vi "IsReadyToKick.vi"(0 "KickToSkill in":refnum<class "KickToSkill.lvclass">, 1 "KickEps":dbl, 2 "KickRange":dbl, 5 "Game":refnum<class "Game.lvclass">, 7 "Target":dbl[](array[numeric]), 9 "Robot":refnum<class "Robot.lvclass">, 11 "error in (no error)":errorcluster, 12 "MinDistToKick":dbl, 13 "KickingAngle":dbl, 14 "DistToKickingAngle":dbl) -> (4 "KickToSkill out":refnum<class "KickToSkill.lvclass">, 6 "CanKick?":bool, 15 "error out":errorcluster)   [LabVIEW 2020, in "KickToSkill.lvclass"]
uses:
  KickToSkill.lvclass
  Game_class/Game.lvclass
  Robot_class/Robot.lvclass
  Utilities_class/Utilities.lvclass
  Object_class/Object.lvclass/Object.ctl
  Robot_class/Robot.lvclass/Robot.ctl
  Game_class/Game.lvclass/Game.ctl
  <vilib>/Analysis/coordinate.llb/2D Cartesian Coordinate Rotation (Scalar).vi
  Game_class/Read BallRef.vi
  Object_class/Read x.vi
  Object_class/Read y.vi
  Robot_class/Read orientation.vi
  Ball_class/Ball.lvclass
  <vilib>/Analysis/NI_AALPro.lvlib
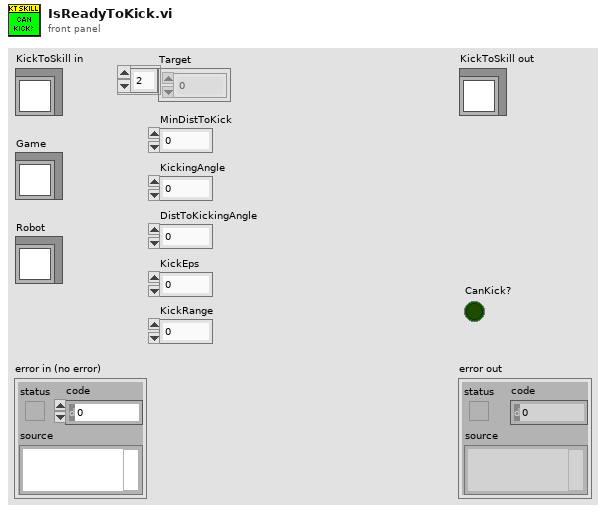
[diagram p1: front panel]
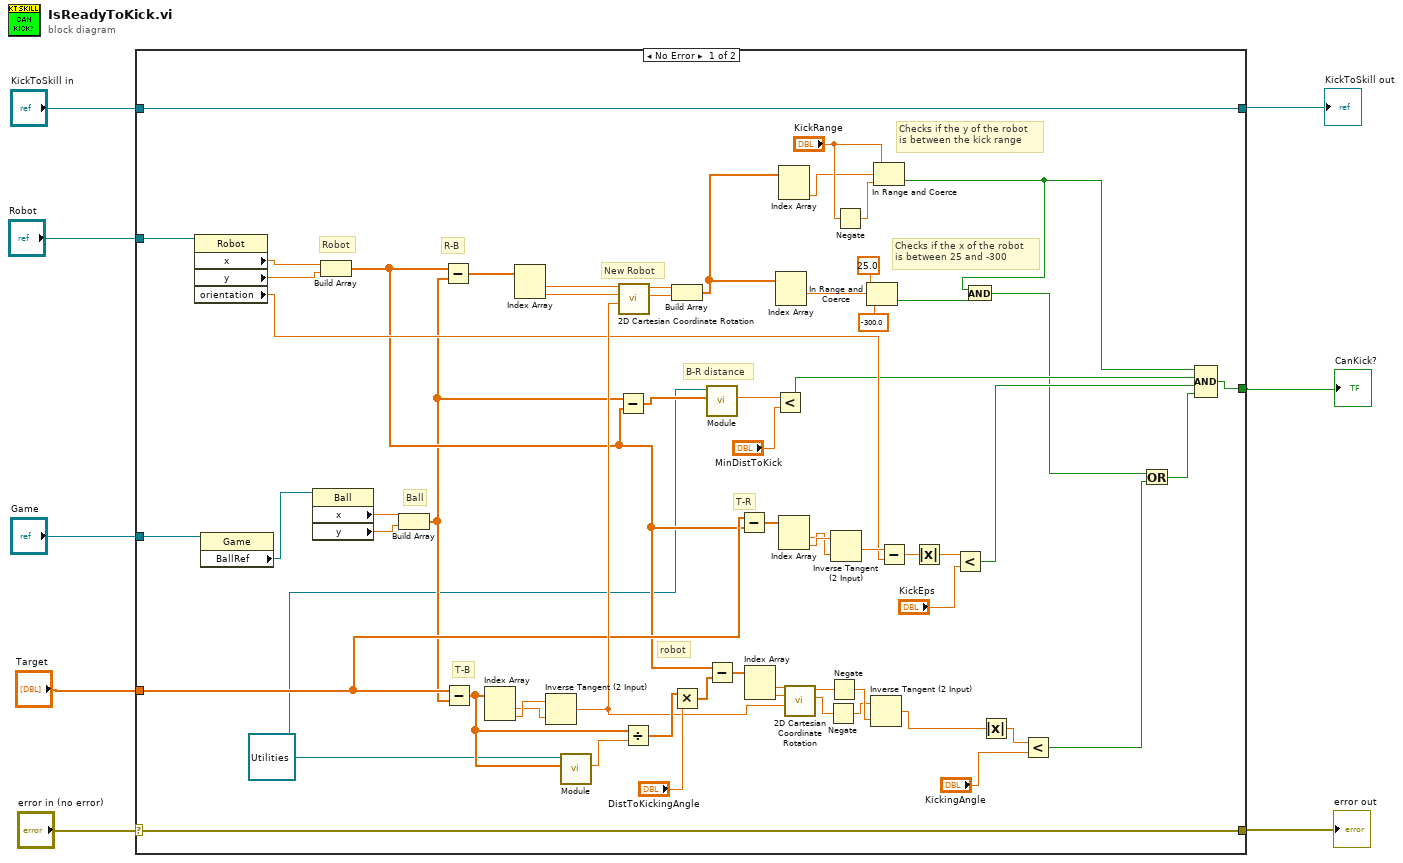
[diagram p0: block diagram]
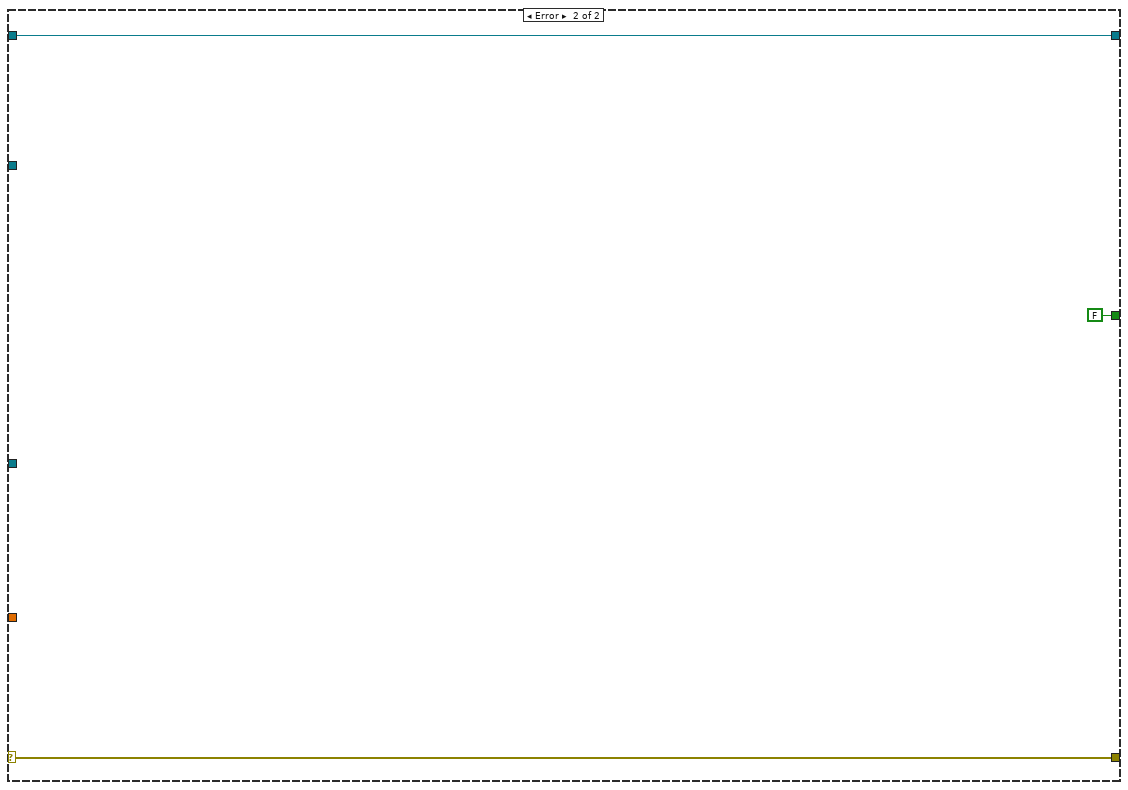
[diagram p2: hidden frame]
diagram:
  n1 = case shown="No Error" "error in (no error)" {
    selector: "error in (no error)" -> [w69 w73]
    tunnel: [w69 w73] -> w7
    tunnel: [w70 w72] -> w5
    tunnel: "KickToSkill in" -> [w70 w72]
    tunnel: "Robot" -> [w68 _]
    tunnel: "Game" -> [w65 _]
    tunnel: "Target" -> [w29 _]
    tunnel: [w13 FALSE] -> w1
    frame No Error {
      w9 = refnum<class "Utilities.lvclass"> refnum ("Utilities in")
      # "T-R"
      # "B-R distance"
      # "Checks if the x of the robot\nis between 25 and -300"
      # "robot"
      # "Checks if the y of the robot\nis between the kick range"
      # "New Robot"
      # "R-B"
      # "T-B"
      # "Ball"
      # "Robot"
      n2 = property class="Robot"(reference=w68) -> ("x"=w67:dbl, "y"=w66:dbl, "orientation"=w24:dbl)  [unwired: 1 in, 2 out]
      n3 = property class="Game"(reference=w65) -> ("BallRef"=w64:refnum<class "Ball.lvclass">)  [unwired: 1 in, 2 out]
      n4 = property class="Ball"(reference=w64) -> ("x"=w63:dbl, "y"=w62:dbl)  [unwired: 1 in, 2 out]
      n5 = Build Array(w67, w66) -> (w12:dbl[])
      n6 = Build Array(w63, w62) -> (w11:dbl[])
      n7 = Subtract(x=w12, y=w11) -> (x-y=w59:dbl[])
      n8 = Subtract(x=w29, y=w11) -> (x-y=w47:dbl[])
      n9 = Index Array(array=w47) -> (element #1=w60:dbl, element #2=w61:dbl)  [unwired: 2 in]
      n10 = Index Array(array=w59) -> (element #1=w58:dbl, element #2=w57:dbl)  [unwired: 2 in]
      n11 = Inverse Tangent (2 Input)(1:w60, 2:w61) -> (0:w39:dbl)
      n12 = call-dynamic "Module.vi"("2D vector"=w47, "Utilities in"=w9) -> ("Modulo"=w46:dbl)  [unwired: 7 in, 2 out]
      n13 = Subtract(x=w11, y=w12) -> (x-y=w10:dbl[])
      n14 = call-poly <vilib>:"2D Cartesian Coordinate Rotation.vi"("theta"=w39, "y"=w57, "x"=w58) -> ("y out"=w55:dbl, "x out"=w56:dbl)  [unwired: 6 in, 1 out]
      n15 = Divide(x=w47, y=w46) -> (x/y=w45:dbl[])
      n16 = Build Array(w56, w55) -> (w50:dbl[])
      n17 = Multiply(x=w45, y="DistToKickingAngle") -> (x*y=w43:dbl[])
      n18 = call-dynamic "Module.vi"("2D vector"=w10, "Utilities in"=w9) -> ("Modulo"=w31:dbl)  [unwired: 7 in, 2 out]
      n19 = Subtract(x=w12, y=w43) -> (x-y=w42:dbl[])
      n20 = Subtract(x=w29, y=w12) -> (x-y=w28:dbl[])
      n21 = Index Array(array=w42) -> (element #1=w41:dbl, element #2=w40:dbl)  [unwired: 2 in]
      n22 = Less?(x=w31, y="MinDistToKick") -> (x < y?=w20:bool)
      n23 = Index Array(array=w50) -> (element #1=w51:dbl)  [unwired: 2 in, 1 out]
      n24 = Index Array(array=w50) -> (element #2=w52:dbl)  [unwired: 2 in, 1 out]
      n25 = Index Array(array=w28) -> (element #1=w26:dbl, element #2=w27:dbl)  [unwired: 2 in]
      n26 = call-poly <vilib>:"2D Cartesian Coordinate Rotation.vi"("theta"=w39, "y"=w40, "x"=w41) -> ("y out"=w36:dbl, "x out"=w38:dbl)  [unwired: 6 in, 1 out]
      n27 = Negate(x=w36) -> (-x=w35:dbl)
      n28 = Negate(x=w38) -> (-x=w37:dbl)
      n29 = Inverse Tangent (2 Input)(1:w26, 2:w27) -> (0:w25:dbl)
      n30 = Negate(x="KickRange") -> (-x=w54:dbl)
      n31 = In Range and Coerce(upper limit=25.0, x=w51, lower limit=-300.0) -> (In Range?=w16:bool)  [unwired: 1 out]
      n32 = Inverse Tangent (2 Input)(1:w37, 2:w35) -> (0:w34:dbl)
      n33 = In Range and Coerce(upper limit="KickRange", x=w52, lower limit=w54) -> (In Range?=w15:bool)  [unwired: 1 out]
      n34 = Subtract(x=w25, y=w24) -> (x-y=w23:dbl)
      n35 = Absolute Value(x=w23) -> (abs(x)=w22:dbl)
      n36 = Less?(x=w22, y="KickEps") -> (x < y?=w19:bool)
      n37 = And(x=w15, y=w16) -> (x .and. y?=w14:bool)
      n38 = Absolute Value(x=w34) -> (abs(x)=w33:dbl)
      n39 = Less?(x=w33, y="KickingAngle") -> (x < y?=w17:bool)
      n40 = Or(x=w14, y=w17) -> (x .or. y?=w18:bool)
      n41 = Compound Arithmetic op=AND(w15, w20, w19, w18) -> (w13:bool)
    }
    frame Error {
    }
  }
  "error out" <- w7
  "KickToSkill out" <- w5
  "CanKick?" <- w1
